vi "macro_HolDrvController_ExecuteSP.vi"   [LabVIEW 2019, in "Trajectory_Library.lvlib"]
uses:
  Trajectory_Library.lvlib
types:
  T1 = typedef "WPILib_Math.lvlib/PID_TUNING.ctl" = cluster{"Kp":dbl, "Ki":dbl, "Kd":dbl, "MaximumIntegral":dbl, "MinimumIntegral":dbl}
  T2 = typedef "WPILib_Math.lvlib/POSE2D.ctl" = cluster{"TRANSLATION":T3, "ROTATION":T4}
  T3 = typedef "WPILib_Math.lvlib/TRANSLATION2D.ctl" = cluster{"X":dbl, "Y":dbl}
  T4 = typedef "WPILib_Math.lvlib/ROTATION2D.ctl" = cluster{"VALUE":dbl, "COS":dbl, "SIN":dbl}
  T5 = typedef "WPILib_Math.lvlib/PROFILED_PID_CONTROLLER.ctl" = cluster{"Controller":T6, "Goal":T7, "Setpoint":T7, "Constraint":T8}
  T6 = typedef "WPILib_Math.lvlib/PID_CONTROLLER.ctl" = cluster{"Kp":dbl, "Ki":dbl, "Kd":dbl, "Period":dbl, "Max_Integral":dbl, "Min_Integral":dbl, "Max_Input":dbl, "Min_Input":dbl, "Continuous":bool, "PositionError":dbl, "VelocityError":dbl, "PrevError":dbl, "TotalError":dbl, "PositionTolerance":dbl, "VelocityTolerance":dbl, "SetPoint":dbl, "Kf":dbl, "Prev_Deriv":dbl, "Prev_Deriv 2":dbl, "DerivativeFilter":bool, "Min_Output":dbl, "Max_Output":dbl, "Prev_F_P":dbl, "Prev_F_P_2":dbl, "AntiWindupActive":bool, "Measurement":dbl}
  T7 = typedef "WPILib_Math.lvlib/TRAPEZOID_PROFILE_STATE.ctl" = cluster{"Position":dbl, "Velocity":dbl}
  T8 = typedef "WPILib_Math.lvlib/TRAPEZOID_PROFILE_CONSTRAINT.ctl" = cluster{"MaxVelocity":dbl, "MaxAcceleration":dbl}
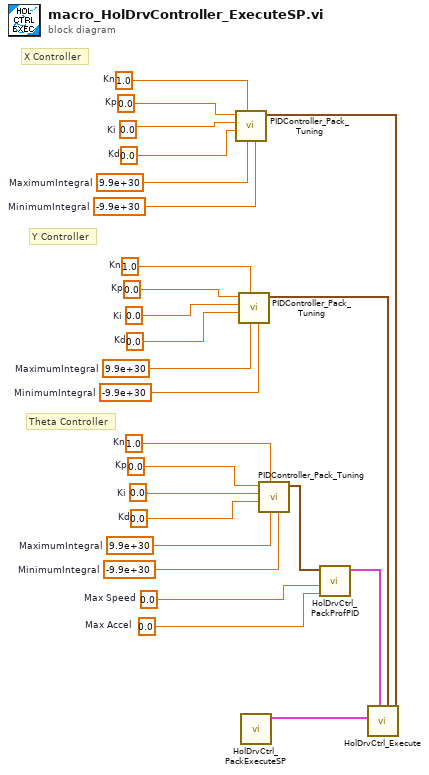
[diagram p0: block diagram]
diagram:
  w17 = 1.0  # Kn
  w14 = 0.0  # Kp
  w5 = 0.0  # Ki
  w4 = 0.0  # Kd
  w3 = 9.9e+30  # MaximumIntegral
  w2 = -9.9e+30  # MinimumIntegral
  w19 = 1.0  # Kn
  w16 = 0.0  # Kp
  w13 = 0.0  # Ki
  w12 = 0.0  # Kd
  w11 = 9.9e+30  # MaximumIntegral
  w10 = -9.9e+30  # MinimumIntegral
  w18 = 1.0  # Kn
  w15 = 0.0  # Kp
  w9 = 0.0  # Ki
  w8 = 0.0  # Kd
  w7 = 9.9e+30  # MaximumIntegral
  w6 = -9.9e+30  # MinimumIntegral
  w20 = 0.0  # Max Accel
  w21 = 0.0  # Max Speed
  # "Theta Controller"
  # "Y Controller"
  # "X Controller"
  n1 = call "PIDController_Pack_Tuning.vi"("MinimumIntegral"=w10, "MaximumIntegral"=w11, "Kn"=w19, "Kd"=w12, "Ki"=w13, "Kp"=w16) -> ("PID Tuning"=w25:T1)  [unwired: 5 in]
  n2 = call "PIDController_Pack_Tuning.vi"("MinimumIntegral"=w6, "MaximumIntegral"=w7, "Kn"=w18, "Kd"=w8, "Ki"=w9, "Kp"=w15) -> ("PID Tuning"=w24:T1)  [unwired: 5 in]
  n3 = call "HolDrvCtrl_PackExecuteSP.vi"() -> ("HolExecuteSP"=w1:cluster{"DesiredPose":T2, "LinearVel":dbl})  [unwired: 11 in]
  n4 = call "PIDController_Pack_Tuning.vi"("MinimumIntegral"=w2, "MaximumIntegral"=w3, "Kn"=w17, "Kd"=w4, "Ki"=w5, "Kp"=w14) -> ("PID Tuning"=w22:T1)  [unwired: 5 in]
  n5 = call "HolDrvCtrl_PackProfPID.vi"("Max Accel"=w20, "Max Speed"=w21, "Theta PID Tuning"=w22) -> ("Theta PID CONTROLLER"=w23:T5)  [unwired: 8 in]
  n6 = call "HolDrvCtrl_Execute.vi"("X PID Tuning"=w25, "Y PID Tuning"=w24, "thetaProfiledPID_CTRL"=w23, "HolExecuteSP"=w1) -> ()  [unwired: 5 in, 3 out]
